vi "Generate Magnification Matrix.vi"(1 "Magnification":dbl) -> (0 "Magnification Matrix":T1)   [LabVIEW 2019, in "Referential.lvclass"]
uses:
  Referential.lvclass
  <vilib>/Analysis/Matrix/Datatypes/RealMatrix.ctl
  <vilib>/Analysis/Matrix/NI_Matrix.lvlib
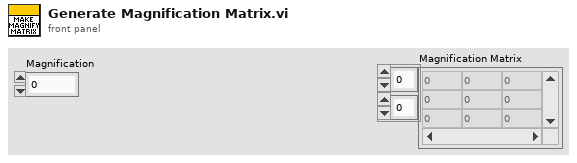
[diagram p1: front panel]
types:
  T1 = typedef "NI_Matrix.lvlib/RealMatrix.ctl" = dbl[][]
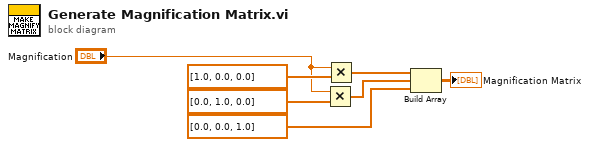
[diagram p0: block diagram]
diagram:
  n1 = Multiply(x="Magnification", y=dbl[] [0.0, 1.0, 0.0] ("element")) -> (x*y=w4:dbl[])
  n2 = Multiply(x="Magnification", y=dbl[] [1.0, 0.0, 0.0] ("element")) -> (x*y=w6:dbl[])
  n3 = Build Array(w6, w4, dbl[] [0.0, 0.0, 1.0] ("element")) -> (→"Magnification Matrix":T1)
